vi "Insert Item.vi"(8 "error in (no error)":errorcluster, 10 "Item":string, 11 "Interactive Tree in":refnum<class "Interactive Tree.lvclass">) -> (0 "error out":errorcluster, 3 "Interactive Tree out":refnum<class "Interactive Tree.lvclass">)   [LabVIEW 2016, in "Interactive Tree.lvclass"]
uses:
  Interactive Tree.lvclass
  Interactive Tree.lvclass/Interactive Tree.ctl
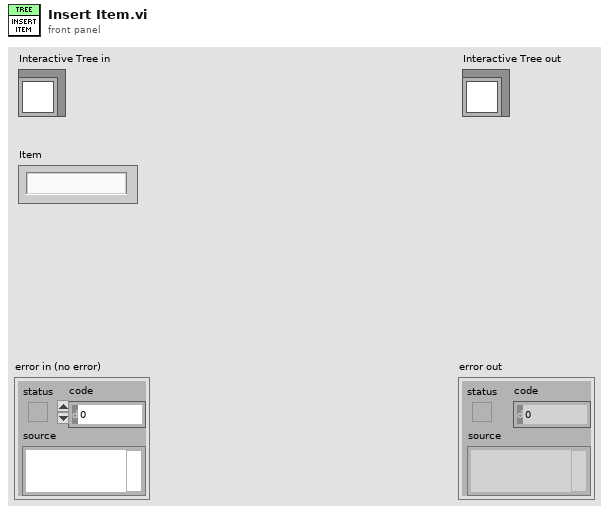
[diagram p1: front panel]
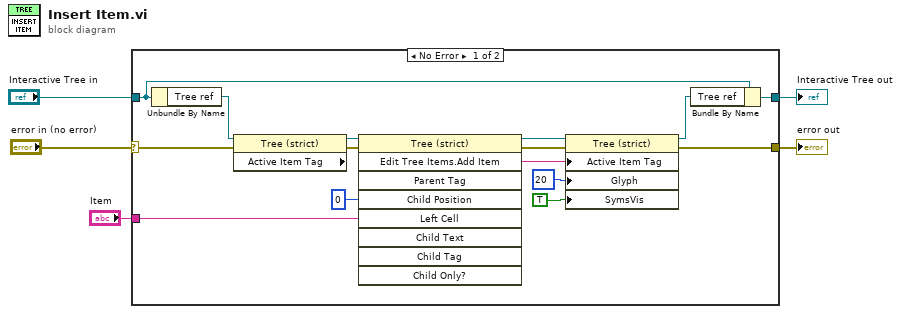
[diagram p0: block diagram]
diagram:
  n1 = case shown="No Error" "error in (no error)" {
    selector: "error in (no error)" -> [w15 w22]
    tunnel: [w6 w22] -> w4
    tunnel: [w14 w21] -> w2
    tunnel: "Interactive Tree in" -> [w20 w21]
    tunnel: "Item" -> [w12 _]
    frame No Error {
      n2 = Unbundle By Name(w20) -> ("Tree ref"=w19:refnum<vi>)
      n3 = property class="Tree (strict)" props=["Active Item Tag"](reference=w19, error in=w15) -> (reference out=w18:refnum<vi>, error out=w17:errorcluster)  [unwired: 1 out]
      n4 = invoke class="Tree (strict)" method="Edit Tree Items.Add Item"(reference=w18, error in=w17, "Child Position"=0, "Left Cell"=w12) -> (reference out=w13:refnum<vi>, error out=w7:errorcluster, "Edit Tree Items:Add Item"=w10:string)  [unwired: 5 in, 6 out]
      n5 = property class="Tree (strict)"(reference=w13, error in=w7, "Active Item Tag"=w10, "Glyph"=20 ("Active Item:Symbol Index"), "SymsVis"=TRUE ("Visible Items:Symbols Visible")) -> (reference out=w11:refnum<vi>, error out=w6:errorcluster)
      n6 = Bundle By Name(cluster=w20, "Tree ref"=w11) -> (w14:refnum<class "Interactive Tree.lvclass">)
    }
    frame Error {
    }
  }
  "error out" <- w4
  "Interactive Tree out" <- w2
